vi "add_uint32.vi"   [LabVIEW 2013]
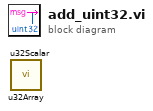
[diagram p0: block diagram]
diagram:
  n1 = call "u32Array.vi"() -> ()  [unwired: 5 in, 1 out]
  n2 = call "u32Scalar.vi"() -> ()  [unwired: 5 in, 1 out]
